vi "Configure Scale Advanced.vi"(7 "Percent Reference (0)":dbl, 8 "error in (no error)":errorcluster, 9 "Offset (0)":dbl, 10 "Gain (1)":dbl=1.0, 11 "VISA resource name":refnum<visa-resource-name>) -> (0 "error out":errorcluster, 3 "VISA resource name out":refnum<visa-resource-name>)   [LabVIEW 2020, in "Agilent 3446X Series.lvlib"]
doc: "Configures advanced scale settings. Used for the \"PCT\" and \"Scale\" scaling functions.\n\n<B>Note(s):</B>\nThis vi is not supported for EDU34450A model.\nThis VI applies only to ACV and DCV measurement functions."
uses:
  Agilent 3446X Series.lvlib
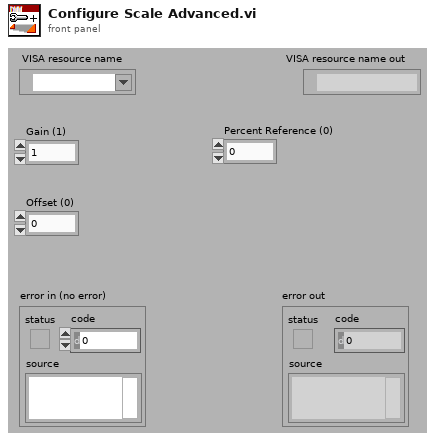
[diagram p1: front panel]
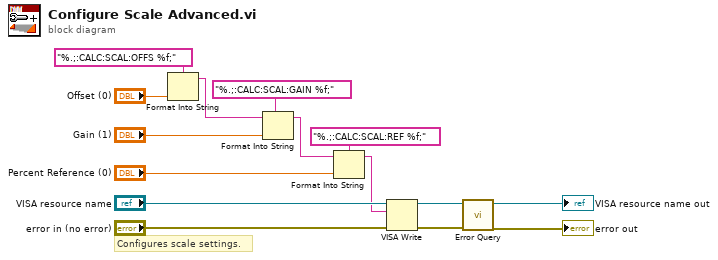
[diagram p0: block diagram]
diagram:
  # "Configures scale settings."
  n1 = Format Into String(format string="%.;:CALC:SCAL:OFFS %f;", "Offset (0)") -> (resulting string=w7:string)  [unwired: 2 in, 1 out]
  n2 = Format Into String(format string="%.;:CALC:SCAL:GAIN %f;", initial string=w7, "Gain (1)") -> (resulting string=w4:string)  [unwired: 1 in, 1 out]
  n3 = Format Into String(format string="%.;:CALC:SCAL:REF %f;", initial string=w4, "Percent Reference (0)") -> (resulting string=w1:string)  [unwired: 1 in, 1 out]
  n4 = VISA Write(VISA resource name="VISA resource name", write buffer=w1, error in (no error)="error in (no error)") -> (VISA resource name out=w13:refnum<visa-resource-name>, error out=w12:errorcluster)  [unwired: 1 out]
  n5 = call "Error Query.vi"("error in (no error)"=w12, "VISA resource name"=w13) -> ("error out"=→"error out":errorcluster, "VISA resource name out"=→"VISA resource name out":refnum<visa-resource-name>)  [unwired: 8 out]
